vi "ScanEngineModeFPGA.vi"() -> ()   [LabVIEW 2017]
uses:
  <vilib>/eio/EIONode/EIONode.xnode
  <vilib>/rvi/eio/common/nirviEmuTemplateMethod_errors.vi
panel:
  out "Chassis Temperature":sgl
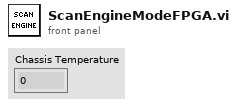
[diagram p1: front panel]
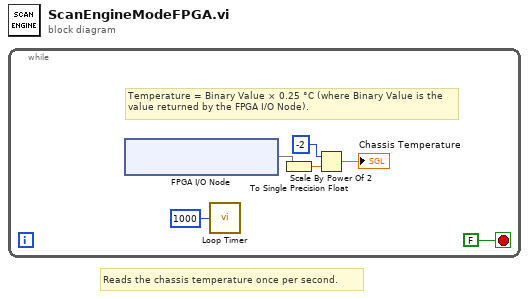
[diagram p0: block diagram]
diagram:
  # "Reads the chassis temperature once per second."
  n1 = while {
    stop <- FALSE stop-if-true
    # "Temperature = Binary Value × 0.25 °C (where Binary Value is the value returned by the FPGA I/O Node)."
    n2 = xnode "FPGA I/O Node"() -> ("Chassis Temperature"=w3)  [unwired: 1 in, 1 out]
    n3 = call "Loop Timer"("Count(mSec)"=u32 1000) -> ()  [unwired: 1 out]
    n4 = To Single Precision Float(number=w3) -> (single precision float=w5:sgl)
    n5 = Scale By Power Of 2(n=i16 -2, x=w5) -> (x*2^n=→"Chassis Temperature":sgl)
  }
